vi "group Bulk Write Tx Packet.vi"(8 "error in (no error)":errorcluster, 11 "group_num":i32) -> (0 "error out":errorcluster)   [LabVIEW 2018, in "labview.lvlib"]
doc: "WINDECLSPEC void groupBulkWriteTxPacket (int group_num);"
uses:
  labview.lvlib
  dxl_x86_c.dll
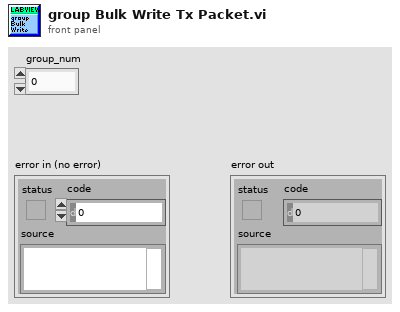
[diagram p1: front panel]
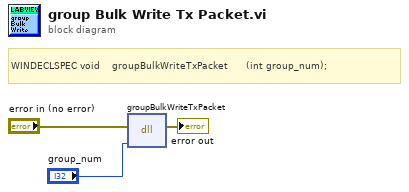
[diagram p0: block diagram]
diagram:
  # "WINDECLSPEC void    groupBulkWriteTxPacket      (int group_num);"
  n1 = dll-call lib="C:/Users/joaos/OneDrive/Documents/[PhD]/Project Omnidirectional Vehicle/Vanes/LabView_code/joaoandthethreestands/DynamixelSDK-3.7.31/labview/new_compilation/dxl_x86_c.*" fn="groupBulkWriteTxPacket"(error in="error in (no error)", "group_num"="group_num") -> (error out=→"error out":errorcluster)  [unwired: 4 in, 1 out]
